vi "Groups.vi"(7 "Type":T9(ring), 10 "Channel Group":T8 {"Holding Registers"."Mapping"."VS Reference" format="%.0x"; "Input Registers"."Mapping"."VS Reference" format="%.0x"; "Discrete Inputs"."Mapping"."VS Reference" format="%.0x"; "Coils"."Mapping"."VS Reference" format="%.0x"}, 11 "Item Ref in":T1 format="%.0x") -> (0 "Engine Group Names":string[](array[string]), 1 "Config Groups":T2[](array[typedef]) {"Channel Data"."Mapping"."VS Reference" format="%.0x"}, 2 "Engine Groups":T10(array[cluster]) {"VS Refs" format="%.0x"}, 3 "Item Ref out":T1 format="%.0x")   [LabVIEW 2021, in "Modbus Master System Explorer.lvlib"]
uses:
  Modbus Master System Explorer.lvlib
  <vilib>/NI VeriStand/Custom Device API/Custom Device Item Ref.ctl
  Shared/Controls/Data Model/Channel Data.ctl
  Shared/Controls/Data Model/Channel.ctl
  Modbus Type.ctl
  <vilib>/NI VeriStand/Custom Device API/Custom Device Channel Type.ctl
  Shared/Controls/Data Model/Mapping.ctl
  Shared/Controls/Data Model/DataType.ctl
  Engine/SubVIs/Bulk Data Access.ctl
  <vilib>/NI VeriStand/Custom Device API/Custom Device API.lvlib
  Shared/Modbus Master Shared.lvlib
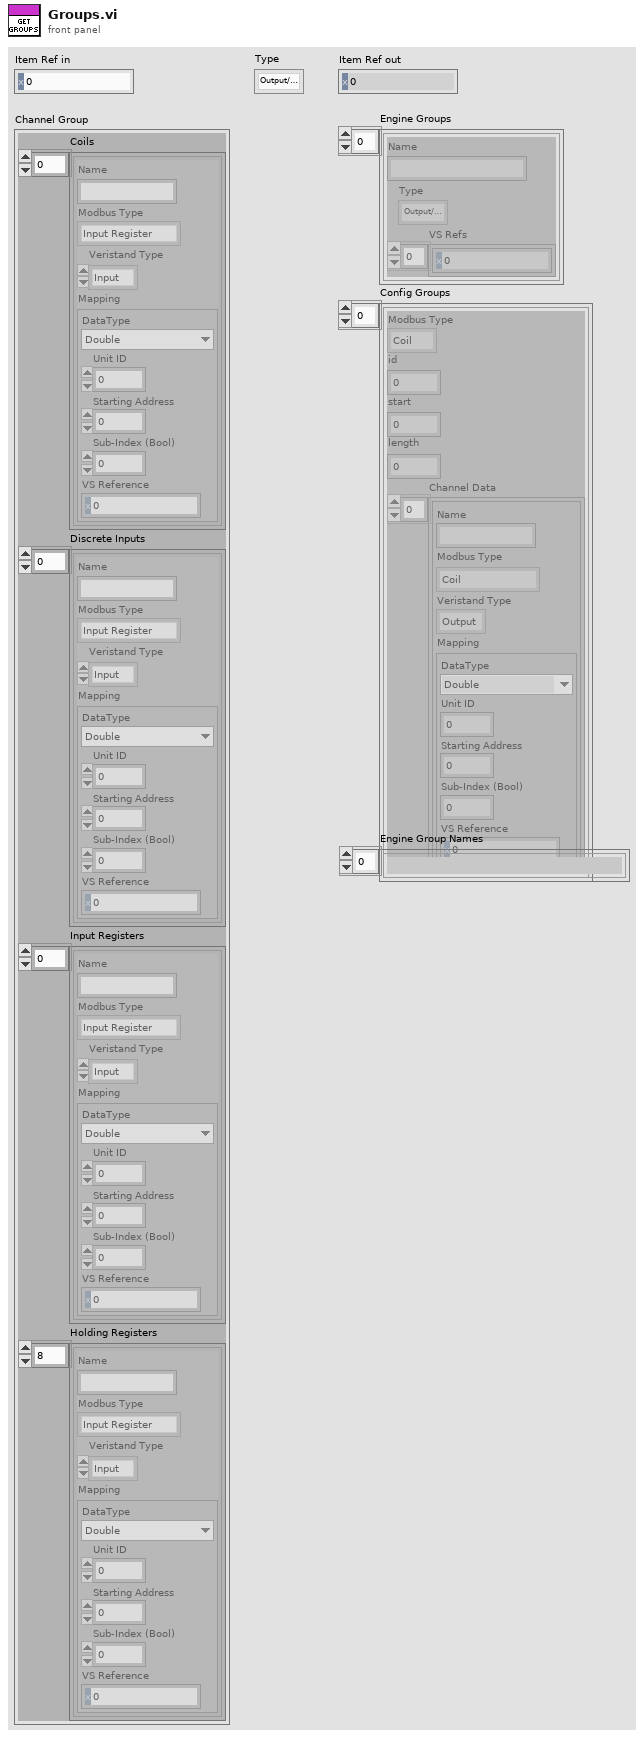
[diagram p1: front panel]
types:
  T1 = typedef "Custom Device API.lvlib/Custom Device Item Ref.ctl" = u64
  T2 = typedef "Modbus Master Shared.lvlib/Bulk Data Access.ctl" = cluster{"Modbus Type":T3, "id":u8, "start":u16, "length":u16, "Channel Data":T4[]}
  T3 = typedef "Modbus Master Shared.lvlib/Modbus Type.ctl" = enum16{"Coil", "Discrete Input", "Holding Register", "Input Register"}
  T4 = typedef "Modbus Master Shared.lvlib/Channel.ctl" = cluster{"Name":string, "Modbus Type":T3, "Veristand Type":T5, "Mapping":T6}
  T5 = typedef "Custom Device API.lvlib/Custom Device Channel Type.ctl" = enum16{"Input", "Output"}
  T6 = typedef "Modbus Master Shared.lvlib/Mapping.ctl" = cluster{"DataType":T7, "Unit ID":u8, "Starting Address":u16, "Sub-Index (Bool)":u16, "VS Reference":T1}
  T7 = typedef "Modbus Master Shared.lvlib/DataType.ctl" = enum16{"Double", "Single", "I64", "I32", "I16", "I8", "U64", "U32", "U16", "U8", "Boolean"}
  T8 = typedef "Modbus Master Shared.lvlib/Channel Data.ctl" = cluster{"Coils":T4[], "Discrete Inputs":T4[], "Input Registers":T4[], "Holding Registers":T4[]}
  T9 = enum16{"Output/Write", "Input/Read", "Input/ReadWrite"}
  T10 = cluster{"Name":string, "Type":enum16{"Output/Write", "Input/Read", "Input/ReadWrite"}, "VS Refs":T1[]}[]
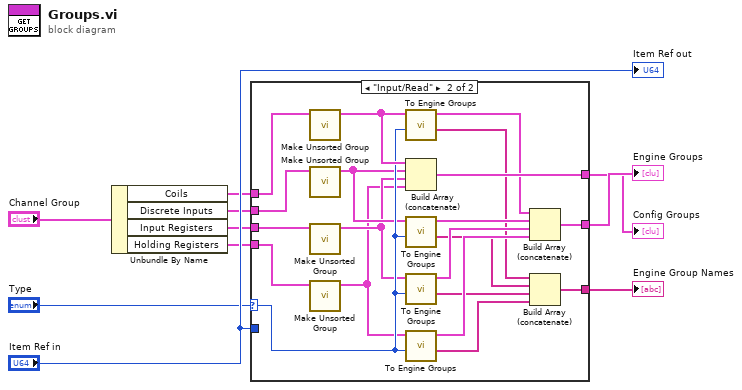
[diagram p0: block diagram]
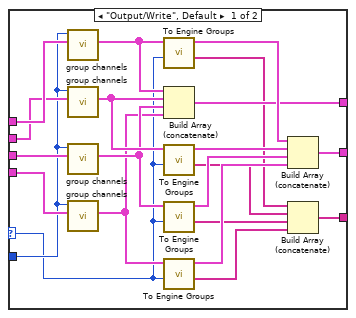
[diagram p2: hidden frame]
diagram:
  n1 = Unbundle By Name("Channel Group") -> ("Coils"=w1:T4[], "Discrete Inputs"=w5:T4[], "Input Registers"=w4:T4[], "Holding Registers"=w3:T4[])
  n2 = case shown="\"Input/Read\"" "Type" {
    selector: "Type" -> [w11 w46]
    tunnel: [w26 w44] -> w10
    tunnel: [w22 w50] -> w9
    tunnel: [w17 w39] -> w8
    tunnel: w1 -> [w16 w38]
    tunnel: w5 -> [w15 w37]
    tunnel: w4 -> [w14 w35]
    tunnel: w3 -> [w13 w33]
    tunnel: "Item Ref in" -> [w12 _]
    frame "Output/Write", Default {
      n3 = call "group channels.vi"("Channels"=w16, "Item Ref in"=w12) -> ("Groups"=w30:T2[])  [unwired: 8 in, 1 out]
      n4 = call "group channels.vi"("Channels"=w15, "Item Ref in"=w12) -> ("Groups"=w25:T2[])  [unwired: 8 in, 1 out]
      n5 = call "group channels.vi"("Channels"=w14, "Item Ref in"=w12) -> ("Groups"=w24:T2[])  [unwired: 8 in, 1 out]
      n6 = call "group channels.vi"("Channels"=w13, "Item Ref in"=w12) -> ("Groups"=w23:T2[])  [unwired: 8 in, 1 out]
      n7 = call "To Engine Groups.vi"("Type"=w11, "Group"=w30) -> ("Names"=w21:string[], "Engine Groups"=w31:T10)  [unwired: 8 in]
      n8 = Build Array (concatenate)(w30, w25, w24, w23) -> (w22:T2[])
      n9 = call "To Engine Groups.vi"("Type"=w11, "Group"=w25) -> ("Names"=w20:string[], "Engine Groups"=w29:T10)  [unwired: 8 in]
      n10 = call "To Engine Groups.vi"("Type"=w11, "Group"=w24) -> ("Names"=w19:string[], "Engine Groups"=w28:T10)  [unwired: 8 in]
      n11 = call "To Engine Groups.vi"("Type"=w11, "Group"=w23) -> ("Names"=w18:string[], "Engine Groups"=w27:T10)  [unwired: 8 in]
      n12 = Build Array (concatenate)(w31, w29, w28, w27) -> (w26:T10)
      n13 = Build Array (concatenate)(w21, w20, w19, w18) -> (w17:string[])
    }
    frame "Input/Read" {
      n14 = call "Make Unsorted Group.vi"("Channels"=w38) -> ("Array"=w51:T2[])  [unwired: 10 in]
      n15 = call "Make Unsorted Group.vi"("Channels"=w37) -> ("Array"=w36:T2[])  [unwired: 10 in]
      n16 = call "Make Unsorted Group.vi"("Channels"=w35) -> ("Array"=w34:T2[])  [unwired: 10 in]
      n17 = call "Make Unsorted Group.vi"("Channels"=w33) -> ("Array"=w32:T2[])  [unwired: 10 in]
      n18 = call "To Engine Groups.vi"("Type"=w46, "Group"=w51) -> ("Names"=w43:string[], "Engine Groups"=w49:T10)  [unwired: 8 in]
      n19 = Build Array (concatenate)(w51, w36, w34, w32) -> (w50:T2[])
      n20 = call "To Engine Groups.vi"("Type"=w46, "Group"=w36) -> ("Names"=w42:string[], "Engine Groups"=w48:T10)  [unwired: 8 in]
      n21 = call "To Engine Groups.vi"("Type"=w46, "Group"=w34) -> ("Names"=w41:string[], "Engine Groups"=w47:T10)  [unwired: 8 in]
      n22 = call "To Engine Groups.vi"("Type"=w46, "Group"=w32) -> ("Names"=w40:string[], "Engine Groups"=w45:T10)  [unwired: 8 in]
      n23 = Build Array (concatenate)(w49, w48, w47, w45) -> (w44:T10)
      n24 = Build Array (concatenate)(w43, w42, w41, w40) -> (w39:string[])
    }
  }
  "Engine Groups" <- w10
  "Config Groups" <- w9
  "Engine Group Names" <- w8
  "Item Ref out" <- "Item Ref in"
